vi "getconfiguration.vi"(8 "error in (no error)":errorcluster, 11 "hObject":i32) -> (0 "error out":errorcluster, 1 "pINumBytes":i32, 2 "pData":u8[](array[numeric]) format="%.0x", 3 "hObject Out":i32)   [LabVIEW 2009]
doc: "this vi reads the configuration from the device\n\n12/21/2010 1.0.0 jyg\n- initial release"
uses:
  NEO VI Example/data/icsneo40.dll
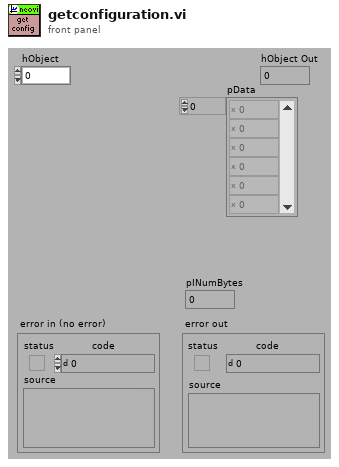
[diagram p1: front panel]
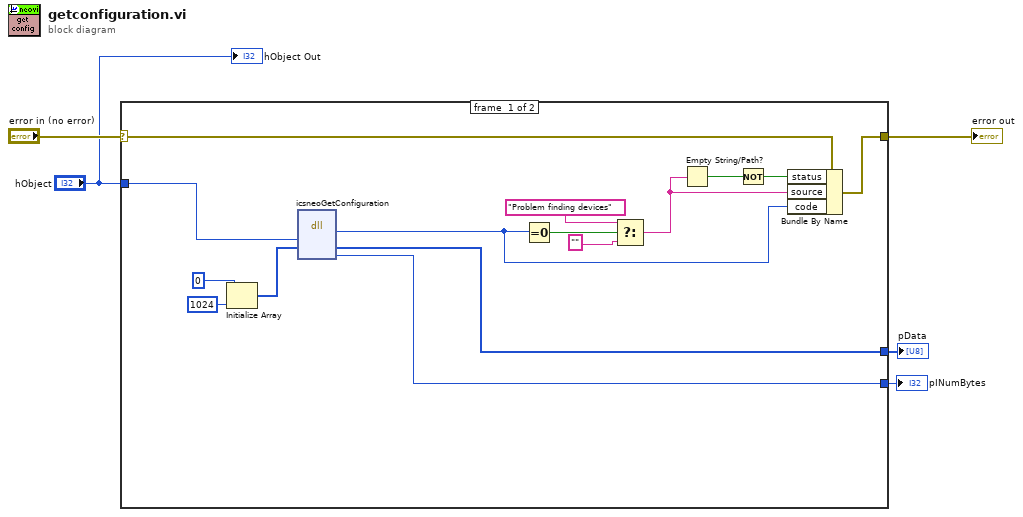
[diagram p0: block diagram]
diagram:
  n1 = case shown="No Error" "error in (no error)" {
    selector: "error in (no error)" -> [w16 w21]
    tunnel: "hObject" -> [w11 _]
    tunnel: [w17 w21] -> w5
    tunnel: [w7 _] -> w2
    tunnel: [w6 _] -> w1
    frame #0 {
      n2 = Initialize Array(u8 0, 1024 ("dimension size")) -> (w8:u8[])
      n3 = dll-call lib="C:/WINDOWS/system32/icsneo40.dll" fn="icsneoGetConfiguration"("hObject"=w11, "pData"=w8) -> ("return type"=w15:i32, "pData"=w7:u8[], "1NumBytes"=w6:i32)  [unwired: 4 in, 3 out]
      n4 = Equal To 0?(x=w15) -> (x = 0?=w14:bool)
      n5 = Select(t="Problem finding devices", s=w14, f="") -> (s? t:f=w13:string)
      n6 = Empty String/Path?(string/path=w13) -> (empty?=w19:bool)
      n7 = Not(x=w19) -> (.not. x?=w18:bool)
      n8 = Bundle By Name(cluster=w16, "status"=w18, "source"=w13, "code"=w15) -> (w17:errorcluster)
    }
    frame #1 {
    }
  }
  "error out" <- w5
  "pINumBytes" <- w1
  "pData" <- w2
  "hObject Out" <- "hObject"
